vi "获取用户UID.vi"(8 "error in (no error)":errorcluster caption="错误输入（无错误）") -> (0 "error out":errorcluster caption="错误输出", 3 "uid":string[](array[string]))   [LabVIEW 2016, in "Alarm interface.lvlib" / "wxpusher.lvlib"]
uses:
  wxpusher.lvlib
  <vilib>/httpClient/LabVIEWHTTPClient.lvlib
panel:
  out "数据":T1
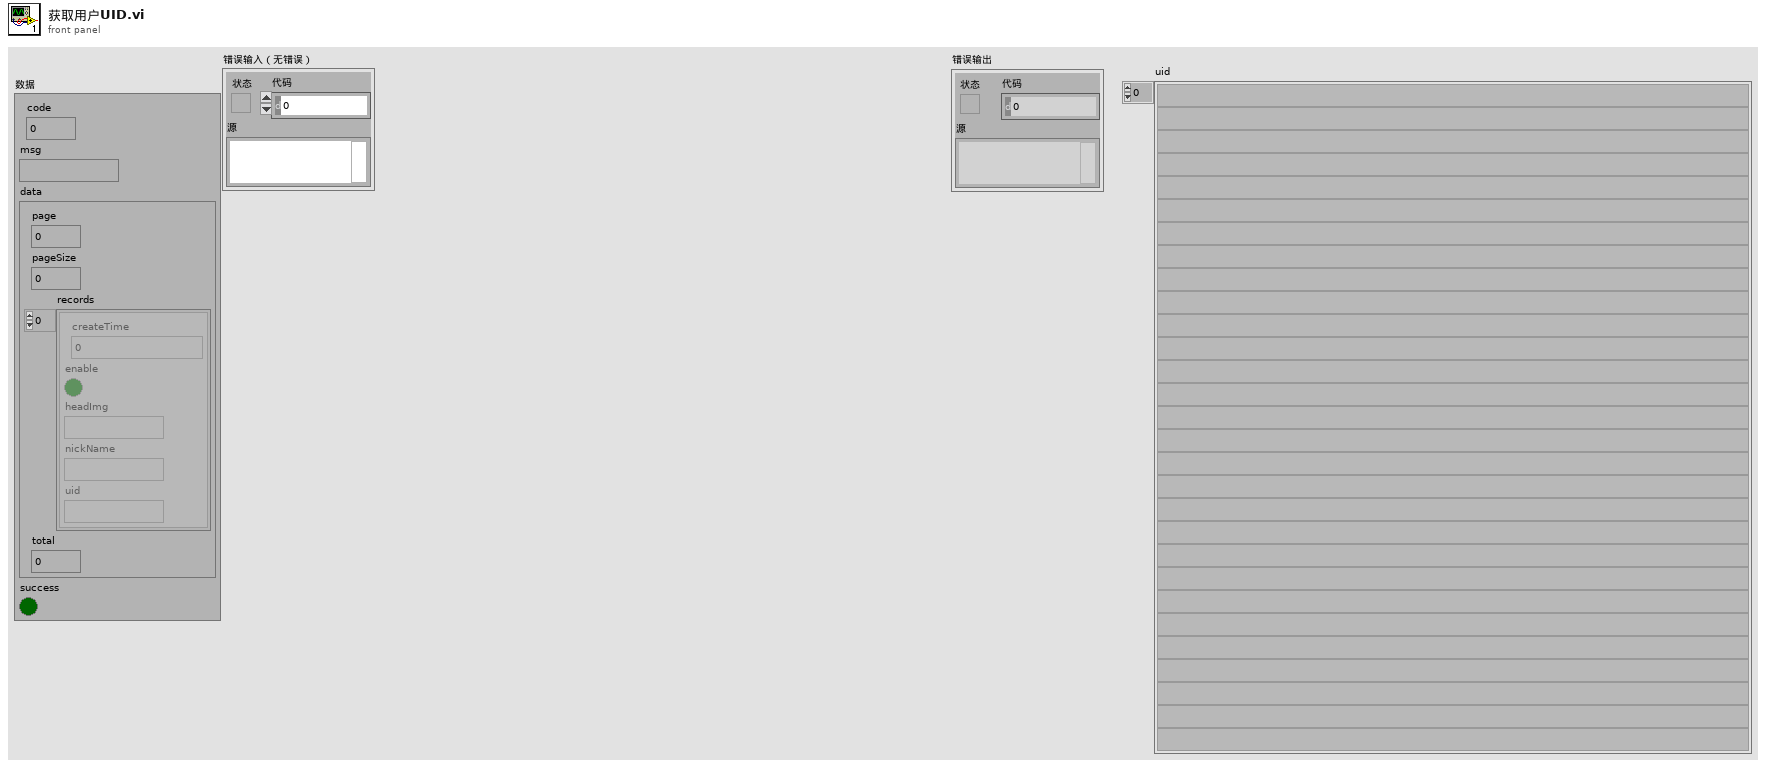
[diagram p1: front panel]
types:
  T1 = cluster{"code":i32, "msg":string, "data":cluster{"page":i32, "pageSize":i32, "records":cluster{"createTime":i32, "enable":bool, "headImg":string, "nickName":string, "uid":string}[], "total":i32}, "success":bool}
  T2 = cluster{"code":i32, "msg":string, "data":cluster{"page":i32, "pageSize":i32, "records":cluster{"createTime":u64, "enable":bool, "headImg":string, "nickName":string, "uid":string}[], "total":i32}, "success":bool}
  T3 = typedef "LabVIEWHTTPClient.lvlib/ClientHandle.ctl" = refnum<k1>
  T4 = cluster{"createTime":u64, "enable":bool, "headImg":string, "nickName":string, "uid":string}[]
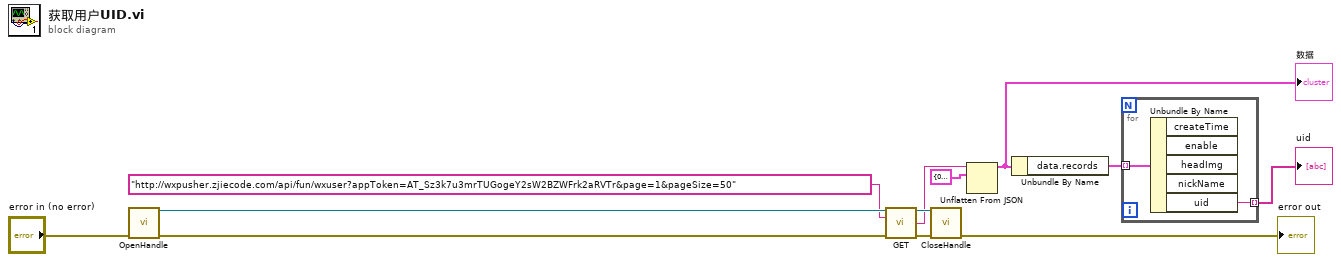
[diagram p0: block diagram]
diagram:
  n1 = call <vilib>:"OpenHandle.vi"("error in (no error)"="error in (no error)") -> ("client handle out"=w10:T3, "error out"=w9:errorcluster)  [unwired: 13 in]
  n2 = call <vilib>:"GET.vi"("client handle"=w10, "url"="http://wxpusher.zjiecode.com/api/fun/wxuser?appToken=AT_Sz3k7u3mrTUGogeY2sW2BZWFrk2aRVTr&page=1&pageSize=50", "error in (no error)"=w9) -> ("client handle out"=w11:T3, "body"=w6:string, "error out"=w12:errorcluster)  [unwired: 9 in, 1 out]
  n3 = call <vilib>:"CloseHandle.vi"("client handle"=w11, "error in (no error)"=w12) -> ("error out"=→"error out":errorcluster)  [unwired: 13 in]
  n4 = Unflatten From JSON(JSON string=w6, type and defaults=T2 {"code"=0, "msg"="", "data"={"page"=0, "pageSize"=0, "records"=[], "total"=0}, "success"=FALSE}) -> (value=w4:T2)  [unwired: 5 in, 1 out]
  "数据" <- w4
  n5 = Unbundle By Name(w4) -> ("data.records"=w7:T4)
  n6 = for {
    tunnel: w7 -> [w14] mode=indexing
    tunnel: [w13] -> w3 mode=indexing
    n7 = Unbundle By Name(w14) -> ("uid"=w13:string)  [unwired: 4 out]
  }
  "uid" <- w3
